vi "Assistant Simple channel example.vi"() -> ()   [LabVIEW 2020]
panel:
  in  "Value":dbl=2.5
  out "Waveform Chart":dynamicdata(graph)
  in  "stop":bool
  out "error out":errorcluster
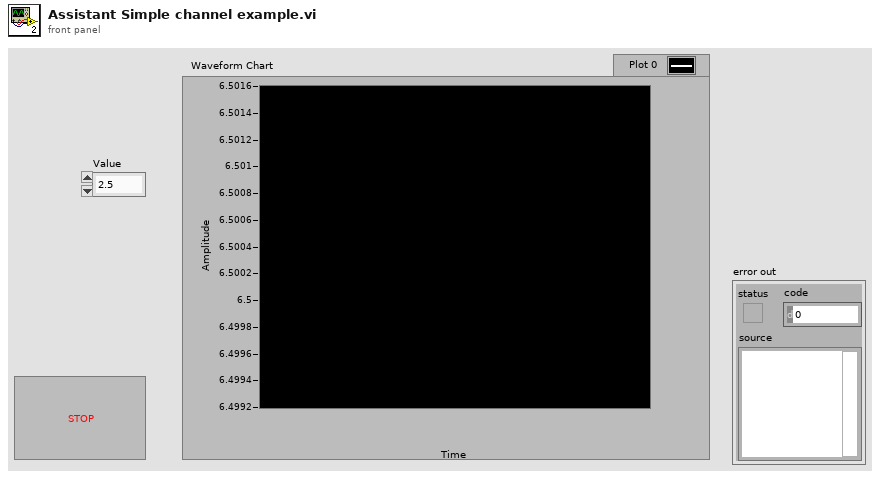
[diagram p1: front panel]
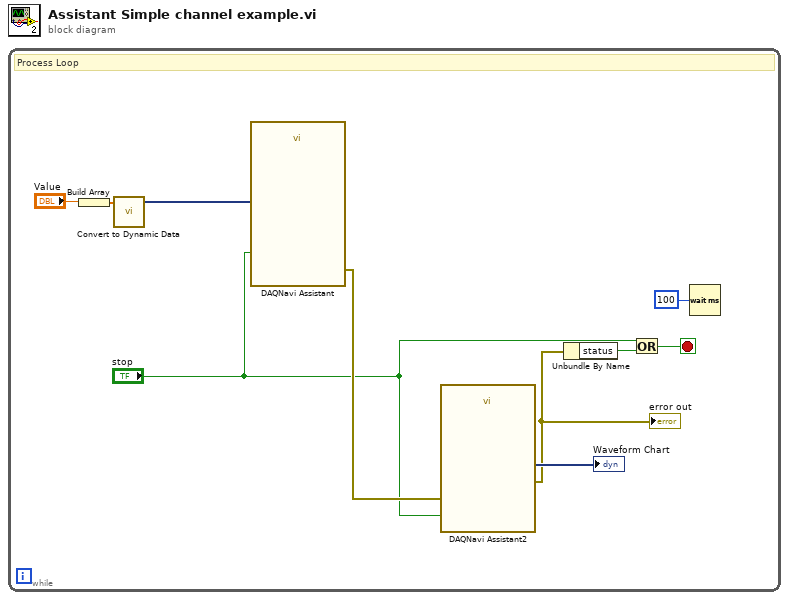
[diagram p0: block diagram]
diagram:
  n1 = while {
    stop <- w9 stop-if-true
    # "Process Loop"
    n2 = Build Array("Value") -> (w1:dbl[])
    n3 = call "Convert to Dynamic Data"("Array"=w1) -> ("Dynamic Data Type"=w6:dynamicdata)  [unwired: 3 out]
    n4 = call "DAQNavi Assistant"("stop(true)"="stop", "data in(DDT)"=w6) -> ("error out"=w4:errorcluster)  [unwired: 2 in, 23 out]
    n5 = call "DAQNavi Assistant2"("error in(no error)"=w4, "stop(true)"="stop") -> ("error out"=w5:errorcluster, "data out(DDT)"=→"Waveform Chart":dynamicdata)  [unwired: 16 out]
    "error out" <- w5
    n6 = Unbundle By Name(w5) -> ("status"=w7:bool)
    n7 = Or(x="stop", y=w7) -> (x .or. y?=w9:bool)
    n8 = Wait (ms)(milliseconds to wait=u32 100) -> ()  [unwired: 1 out]
  }
